vi "Delete Key.vi"(8 "error in":errorcluster, 10 "Key":string, 11 "Config in":refnum<class "Config.lvclass">) -> (0 "error out":errorcluster, 3 "Config out":refnum<class "Config.lvclass">)   [LabVIEW 2023, in "Config.lvlib" / "Config.lvclass"]
uses:
  Config.lvclass
  Config.lvclass/Config.ctl
  <vilib>/Utility/config.llb/NI_LVConfig.lvlib
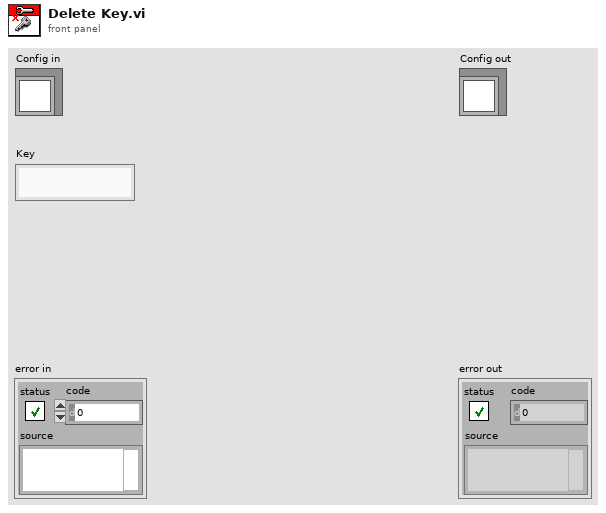
[diagram p1: front panel]
types:
  T1 = typedef "NI_LVConfig.lvlib/Config Data RefNum.ctl" = refnum<k1>
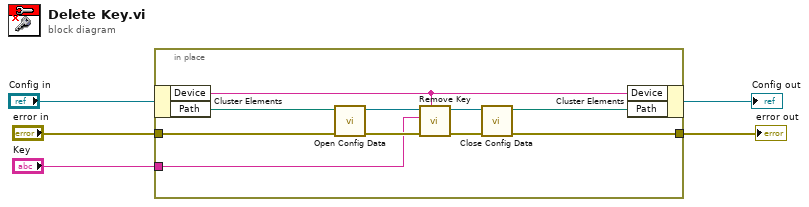
[diagram p0: block diagram]
diagram:
  n1 = in-place {
    in-place-border: [w8] -> w3
    in-place-border: "error in" -> [w7]
    in-place-border: "Key" -> [w6]
    n2 = in-place-cluster #1("Config in") -> ("Device"=w12:string, "Path"=w14:path)
    n3 = call <vilib>:"Open Config Data.vi"("error in (no error)"=w7, "configuration file path"=w14) -> ("error out"=w10:errorcluster, "refnum"=w15:T1)  [unwired: 7 in, 1 out]
    n4 = call <vilib>:"Remove Key.vi"("section"=w12, "error in (no error)"=w10, "key"=w6, "refnum"=w15) -> ("error out"=w11:errorcluster, "refnum out"=w9:T1)  [unwired: 5 in, 1 out]
    n5 = call <vilib>:"Close Config Data.vi"("error in (no error)"=w11, "refnum"=w9) -> ("error out"=w8:errorcluster, "file path"=w13:path)  [unwired: 8 in]
    n6 = in-place-cluster #1("Device"=w12, "Path"=w13) -> (→"Config out":refnum<class "Config.lvclass">)
  }
  "error out" <- w3
